vi "New Analog Reader Actor.vi"(8 "error in (no error)":errorcluster, 9 "Loop Period in ms (10)":u32=10, 10 "DAQmx Task":refnum<k21>, 11 "Analog Reader in":refnum<class "Analog Reader.lvclass">) -> (0 "error out":errorcluster, 3 "Analog Reader out":refnum<class "Analog Reader.lvclass">)   [LabVIEW 2024, in "DAQmx Actor.lvlib" / "Analog Reader.lvclass"]
uses:
  Analog Reader.lvclass
  Analog Reader.lvclass/Analog Reader.ctl
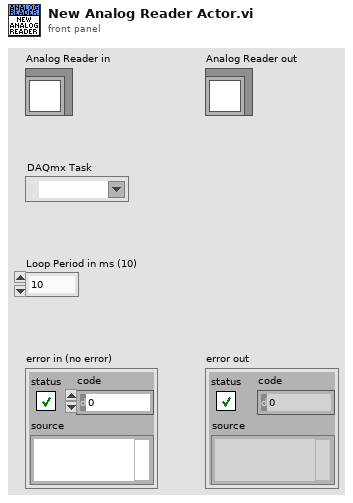
[diagram p1: front panel]
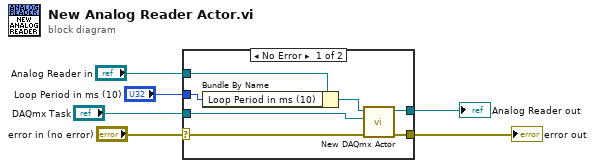
[diagram p0: block diagram]
diagram:
  n1 = case shown="No Error" "error in (no error)" {
    selector: "error in (no error)" -> [w9 w15]
    tunnel: [w8 w15] -> w5
    tunnel: [w7 w14] -> w3
    tunnel: "Analog Reader in" -> [w13 w14]
    tunnel: "Loop Period in ms (10)" -> [w12 _]
    tunnel: "DAQmx Task" -> [w10 _]
    frame No Error {
      n2 = Bundle By Name(cluster=w13, "Loop Period in ms (10)"=w12) -> (w11:refnum<class "Analog Reader.lvclass">)
      n3 = call-dynamic "New DAQmx Actor.vi"("error in (no error)"=w9, "DAQmx Task"=w10, "DAQmx Actor in"=w11) -> ("error out"=w8:errorcluster, "DAQmx Actor out"=w7:refnum<class "Analog Reader.lvclass">)  [unwired: 7 in]
    }
    frame Error {
    }
  }
  "error out" <- w5
  "Analog Reader out" <- w3
